vi "Add Tool.vi"(6 "Ignored":string[](array[string])=["error in"], 8 "error in (no error)":errorcluster, 10 "vi path":path, 11 "server id":i32) -> (0 "error out":errorcluster, 3 "server id out":i32)   [LabVIEW 2025, in "MCP Server.lvlib"]
doc: "Adds a \"tool\" to the MCP server. Tools are functions the LLM can call during a chat response. Tools are SubVIs. Controls on the connector pane of the SubVI are the in- and outputs of a tool. Use \"irgnored\" to hide any control from the LLM. Use the description property of a control to add additional information to the parameter for the LLM. Use the VI description for an overall human understandable description of the function and it's usage. Be precise, but don't write tons of text, this description will cost you tokens."
uses:
  MCP Server.lvlib
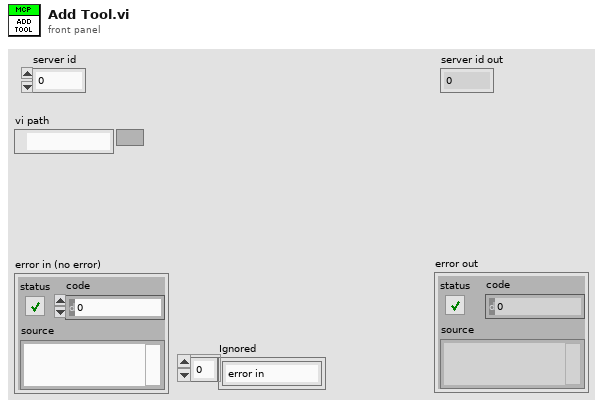
[diagram p1: front panel]
types:
  T1 = typedef "MCP Server.lvlib/Tool Data.ctl" = cluster{"Name":string, "Description":string, "Ignored":string[], "inputs":T2[], "outputs":T3[], "VI Refnum":refnum<vi>}
  T2 = typedef "MCP Server.lvlib/Input Parameter.ctl" = cluster{"name":string, "type":string, "description":string, "required":bool, "raw name":string}
  T3 = typedef "MCP Server.lvlib/Output Parameter.ctl" = cluster{"name":string, "description":string, "type":string, "raw name":string}
  T4 = typedef "MCP Server.lvlib/Server Data.ctl" = cluster{"Name":string, "Description":string, "Tools":T1[], "Parameters":string[][], "Logging Info":T5, "User Events":T6, "Prompts":T7[], "resources":T9[], "HTTP Server":refnum<class "Server.lvclass">}
  T5 = typedef "MCP Server.lvlib/Logging.ctl" = cluster{"Log":string[], "Max Length":i32}
  T6 = typedef "MCP Server.lvlib/User Events.ctl" = cluster{"onError":refnum<user-event>, "onRpc":refnum<user-event>}
  T7 = typedef "MCP Server.lvlib/Prompt Data.ctl" = cluster{"name":string, "description":string, "arguments":T8[], "return terminal name":string, "results description":string, "VI Refnum":refnum<vi>}
  T8 = typedef "MCP Server.lvlib/Prompt Argument.ctl" = cluster{"name":string, "description":string, "required":bool, "raw_name":string}
  T9 = typedef "MCP Server.lvlib/resource data.ctl" = cluster{"uri":string, "name":string, "description":string, "mimeType":string, "file path":path}
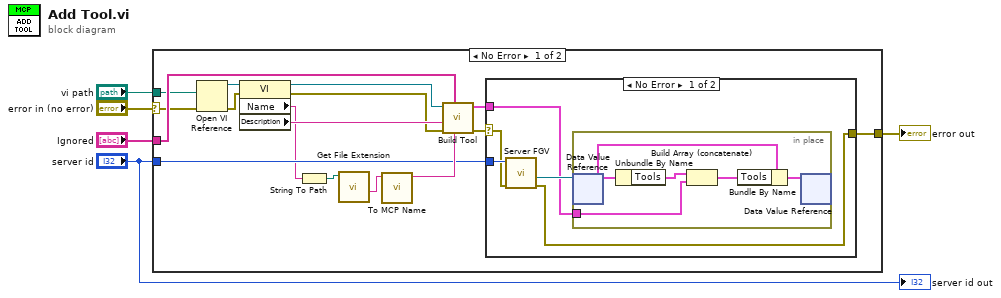
[diagram p0: block diagram]
diagram:
  n1 = case shown="No Error" "error in (no error)" {
    selector: "error in (no error)" -> [w7 w33]
    tunnel: "Ignored" -> [w21 _]
    tunnel: [w14 w33] -> w4
    tunnel: "server id" -> [w13 _]
    tunnel: "vi path" -> [w9 _]
    frame No Error {
      n2 = Open VI Reference(vi path=w9, error in (no error)=w7) -> (vi reference=w16:refnum<vi>, error out=w15:errorcluster)  [unwired: 4 in]
      n3 = property class="VI"(reference=w16, error in=w15) -> (reference out=w6:refnum<vi>, error out=w10:errorcluster, "Name"=w8:string, "Description"=w18:string)
      n4 = String To Path(string=w8) -> (path=w17:path)
      n5 = call <vilib>:"Get File Extension.vi"("file"=w17) -> ("filename without extension"=w19:string)  [unwired: 6 in, 4 out]
      n6 = call "To MCP Name.vi"("unformatted name"=w19) -> ("MCP name"=w20:string)  [unwired: 10 in]
      n7 = call "Build Tool.vi"("String"=w20, "Ignored"=w21, "error in (no error)"=w10, "Description"=w18, "VI Refnum"=w6) -> ("error out"=w12:errorcluster, "array"=w11:T1)  [unwired: 5 in]
      n8 = case shown="No Error" w12 {
        selector: w12 -> [w22 w32]
        tunnel: [w26 w32] -> w14
        tunnel: w13 -> [w25 _]
        tunnel: w11 -> [w23 _]
        frame No Error {
          n9 = call "Server FGV.vi"("error in"=w22, "id"=w25) -> ("error out"=w26:errorcluster, "server reference"=w24:refnum<data-value>)  [unwired: 5 in, 3 out]
          n10 = in-place {
            in-place-border: w23 -> [w27]
            n11 = in-place-dvr #1(w24) -> (w30:T4)  [unwired: 1 out]
            n12 = Unbundle By Name(w30) -> ("Tools"=w31:T1[])
            n13 = Build Array (concatenate)(w31, w27) -> (w29:T1[])
            n14 = Bundle By Name(cluster=w30, "Tools"=w29) -> (w28:T4)
            n15 = in-place-dvr #1(w28) -> ()  [unwired: 2 out]
          }
        }
        frame Error {
        }
      }
    }
    frame Error {
    }
  }
  "error out" <- w4
  "server id out" <- "server id"
